vi "Autocycle v0.4.vi"(7 "Message Queue":refnum<queue>, 8 "error in":errorcluster, 10 "All Para":cluster{"Auto Para":T1, "General Para":T2}={"Auto Para"={"Agitator Delays"=[], "TF Delays"=[], "Insertion Delays"=[], "Cutting Delays"=[], "PF Delays"=[], "Measur. Delays"=[], "Reject Delays"=[1000], "BF Delays"=[1000]}, "General Para"={"Max. Cons."=5.0, "Offset 1"=0.0, "Offset 2"=0.0, "Offset 3"=0.0, "Offset 4"=0.0}}) -> (0 "error out":errorcluster)   [LabVIEW 2017]
doc: "v0.3:\n- Added End Cycle & Stop initiated as different stops\n- Make PF & TF not run on the first iteration"
uses:
  support/Message Queue/Message Cluster.ctl
  Controls/Auto Delays.ctl
  support/Controls/General Para.ctl
  Controls/Auto Times.ctl
  Global Variables/RT GV.vi
  Global Variables/FPGA GV.vi
  <vilib>/Utility/error.llb/Error Cluster From Error Code.vi
  <vilib>/rvi/errors/niLvFpgaAdjustHostInterfaceError.vi
  support/Message Queue/Enqueue Message (Single).vi
  <vilib>/rvi/interface/nirviReadWriteControl/nirviReadWriteControl.xnode
  Controls/FPGA Ref.ctl
  NiFpgaLv.dll
  <vilib>/rvi/interface/Simulation/niFpgaSimulationCallBeginRW.vi
  support/Message Queue/Message Queue.lvlib
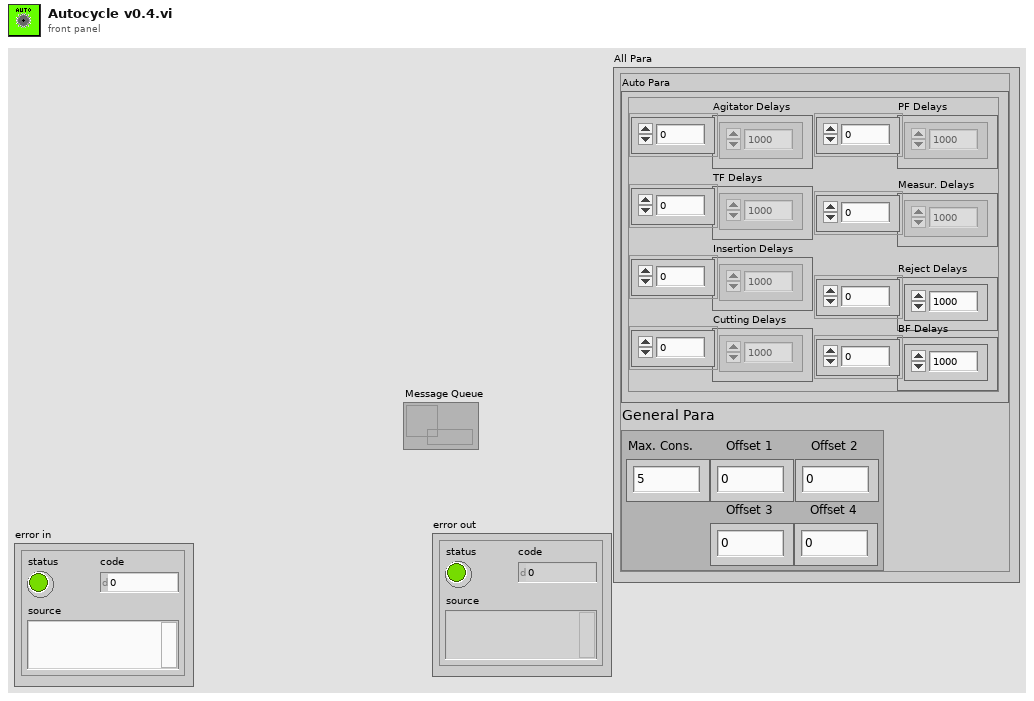
[diagram p1: front panel]
types:
  T1 = typedef "Auto Delays.ctl" = cluster{"Agitator Delays":u32[], "TF Delays":u32[], "Insertion Delays":u32[], "Cutting Delays":u32[], "PF Delays":u32[], "Measur. Delays":dbl[], "Reject Delays":u32[], "BF Delays":u32[]}
  T2 = typedef "General Para.ctl" = cluster{"Max. Cons.":dbl, "Offset 1":dbl, "Offset 2":dbl, "Offset 3":dbl, "Offset 4":dbl}
  T3 = cluster{"Tube Present":bool[], "Output Count":u32}
  T4 = typedef "FPGA Ref.ctl" = refnum<k20>
  T5 = cluster{"TL_Red":bool, "TL_Orange":bool, "TL_Green":bool, "TL_Buzzer":bool, "SOL_Index_Rotary_CW":bool, "SOL_Index_CNVR_Rotary_CCW":bool, "SOL_Index_CNVR_Stopper_Rear":bool, "SOL_Index_CNVR_Output _Separator _Rear":bool, "Bowl Feeder_ ON1":bool, "Pump_CNVR_Motor _ON":bool, "SOL_PC_Gating_CYL_Rear":bool, "SOL_Tube_Feed_Agitatator":bool, "SOL_Tube_Feed_Gating_CYL":bool, "SOL_Insertion _CYL":bool, "SOL_Insertion_Clamp_CYL":bool, "SOL_Cutting_CYL":bool, "SOL_Cutting_Clamp_CYL":bool, "SOL_Insertion_Air_Nozzle":bool, "SOL_Measurement_CYL":bool, "DO1.19":bool, "SOL_Rejection CYL_1":bool, "SOL_Rejection CYL_2":bool, "SOL_Rejection CYL_3":bool, "SOL_Rejection CYL_4":bool, "Bowl Feeder_ON2":bool, "SOL_BF_BlowerON":bool, "SOL_BF1_Track1":bool, "SOL_BF1_Track2":bool, "SOL_BF2_Track1":bool, "SOL_BF2_Track2":bool, "DO1.30":bool, "DO1.31":bool}
  T6 = typedef "Auto Times.ctl" = cluster{"Index Time":u32, "TF Time":u32, "Insertion Time":u32, "Cutting Time":u32, "PF Time":u32, "Meas. Time":u32, "Reject Time":u32}
  T7 = cluster{"Reject 1":bool, "Reject 2":bool, "Reject 3":bool, "Reject 4":bool}
  T8 = cluster{"Tube Present":bool[], "Parts Count":u32}
  T9 = cluster{"seconds since 1Jan1904":timestamp, "Auto Times":T6, "Tube Present":bool[], "Reject Pallets":cluster{"Reject 1":bool, "Reject 2":bool, "Reject 3":bool, "Reject 4":bool}, "Measurements":cluster{"1":dbl, "2":dbl, "3":dbl, "4":dbl}}
  T10 = typedef "Auto Stats.ctl" = cluster{"Time-Stamp":timestamp, "Auto Times":T6, "Measurements":cluster{"1":dbl, "2":dbl, "3":dbl, "4":dbl}, "Outputs":cluster{"Good Parts":u32, "Reject Parts":u32}, "Cycle Time":dbl, "Remarks":string}
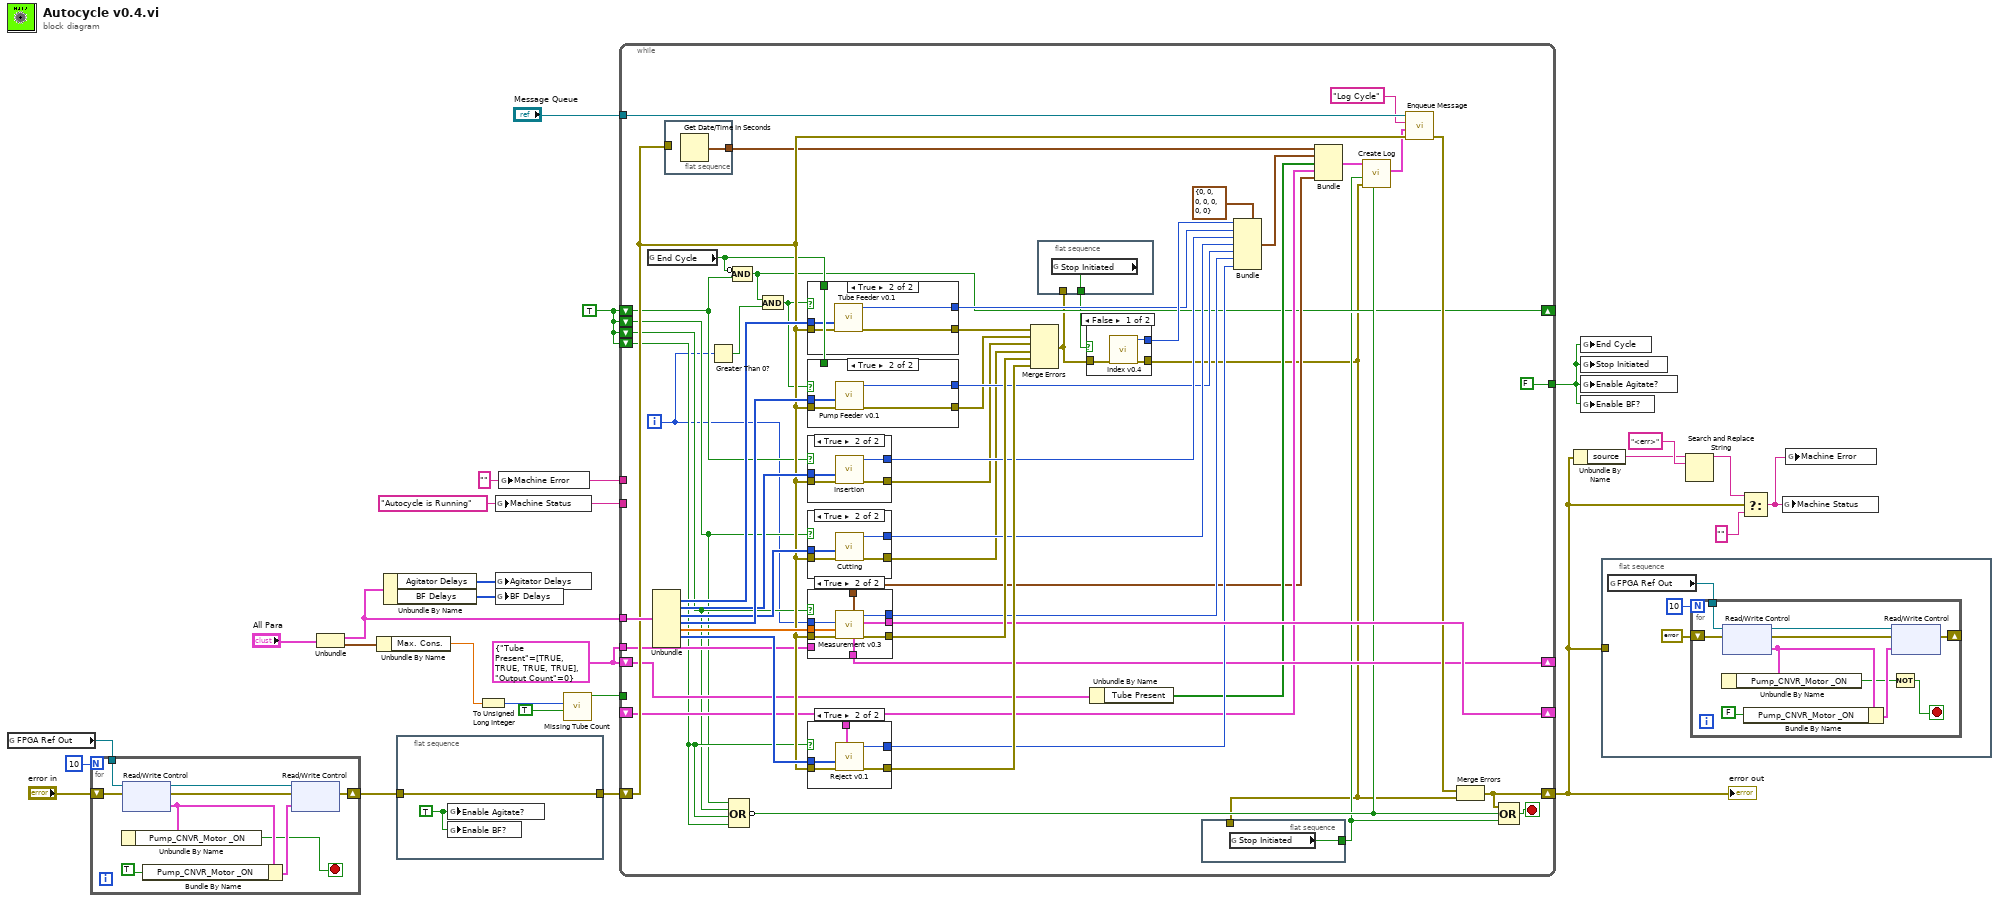
[diagram p0: block diagram]
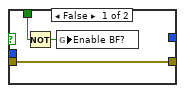
[diagram p3: hidden frame]
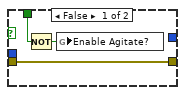
[diagram p6: hidden frame]
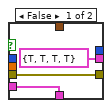
[diagram p8: hidden frame]
diagram:
  w13 = T3 {"Tube Present"=[TRUE, TRUE, TRUE, TRUE], "Output Count"=0} ("Part Count")
  w14 = "" ("Machine Error")
  w21 = "Autocycle is Running" ("Machine Status")
  w7 = TRUE
  n1 = global read "FPGA GV.vi" "FPGA Ref Out"() -> (w24:T4)
  n2 = for {
    N: 10 -> [_]
    tunnel: w24 -> [w35]
    shift-right: [w29] -> w10
    shift-left: "error in" -> [w30]
    stop <- w27 stop-if-true
    n3 = xnode "Read/Write Control"("FPGA VI Reference In"=w35, "error in"=w30) -> ("FPGA VI Reference Out"=w31:T4, "error out"=w32:errorcluster, "DO 1"=w28:T5)
    n4 = Unbundle By Name(w28) -> ("Pump_CNVR_Motor _ON"=w27:bool)
    n5 = Bundle By Name(cluster=w28, "Pump_CNVR_Motor _ON"=TRUE) -> (w34:T5)
    n6 = xnode "Read/Write Control"("FPGA VI Reference In"=w31, "error in"=w32, "DO 1"=w34) -> ("error out"=w29:errorcluster)  [unwired: 1 out]
  }
  n7 = Unbundle("All Para") -> ("Auto Para"=w4:T1, "General Para"=w3:T2)
  n8 = Unbundle By Name(w3) -> ("Max. Cons."=w2:dbl)
  n9 = Unbundle By Name(w4) -> ("Agitator Delays"=w26:u32[], "BF Delays"=w25:u32[])
  n10 = flat-sequence {
    tunnel: [w37] -> w9
    tunnel: w10 -> [w37]
    frame #0 {
      w36 = TRUE ("Enable Agitate?")
      n11 = global write "RT GV.vi" "Enable Agitate?"(w36) -> ()
      n12 = global write "RT GV.vi" "Enable BF?"(w36) -> ()
    }
  }
  n13 = To Unsigned Long Integer(number=w2) -> (unsigned 32bit integer=w1:u32)
  n14 = global write "RT GV.vi" "Machine Status"(w21) -> ()
  n15 = global write "RT GV.vi" "Agitator Delays"(w26) -> ()
  n16 = global write "RT GV.vi" "BF Delays"(w25) -> ()
  n17 = global write "RT GV.vi" "Machine Error"(w14) -> ()
  n18 = call "Missing Tube Count.vi"("ResetMT?"=TRUE, "Max Successive"=w1) -> ("Boolean"=w11:bool)  [unwired: 9 in]
  n19 = while {
    tunnel: w4 -> [w86]
    shift-right: [w63] -> w19
    shift-left: w9 -> [w64]
    shift-right: [w80] -> _
    shift-left: _ -> [w54]
    shift-right: [w45] -> _
    shift-left: w7 -> [w46]
    shift-left: w7 -> [w47]
    shift-left: w7 -> [w48]
    shift-left: w7 -> [w49]
    tunnel: "Message Queue" -> [w70]
    tunnel: [FALSE] -> w6
    tunnel: w21 -> [_]
    tunnel: w14 -> [_]
    shift-right: [w57] -> _
    shift-left: w13 -> [w56]
    tunnel: w13 -> [w58]
    tunnel: w11 -> [_]
    i -> [w41]
    stop <- w79 stop-if-true
    n20 = global read "RT GV.vi" "End Cycle"() -> (w50:bool)
    n21 = Unbundle(w86) -> ("TF Delays"=w89:u32[], "Insertion Delays"=w88:u32[], "Cutting Delays"=w87:u32[], "PF Delays"=w90:u32[], "Measur. Delays"=w84:dbl[], "Reject Delays"=w82:u32[])  [unwired: 2 out]
    n22 = flat-sequence {
      tunnel: w64 -> [_]
      tunnel: [w97] -> w60
      frame #0 {
        n23 = Get Date/Time In Seconds() -> (seconds since 1Jan1904=w97:timestamp)
      }
    }
    n24 = Greater Than 0?(x=w41) -> (x > 0?=w43:bool)
    n25 = Compound Arithmetic op=OR(w47, w48, w49, w49) -> (invert w52:bool)
    n26 = Compound Arithmetic op=AND(invert w50, w46) -> (w45:bool)
    n27 = Compound Arithmetic op=AND(w45, w43) -> (w44:bool)
    n28 = case shown="True" w44 {
      tunnel: w64 -> [w117 w121]
      tunnel: [w117 w120] -> w85
      tunnel: w89 -> [_ w119]
      tunnel: [_ w118] -> w77
      tunnel: w50 -> [w116 _]
      frame False {
        n29 = Not(x=w116) -> (.not. x?=w115:bool)
        n30 = global write "RT GV.vi" "Enable Agitate?"(w115) -> ()
      }
      frame True {
        n31 = call "Tube Feeder v0.1.vi"("error in (no error)"=w121, "TF Para"=w119) -> ("error out"=w120:errorcluster, "TF Time"=w118:u32)  [unwired: 8 in]
      }
    }
    n32 = case shown="True" w44 {
      tunnel: w64 -> [w100 w104]
      tunnel: [w100 w103] -> w66
      tunnel: w90 -> [_ w102]
      tunnel: [_ w101] -> w74
      tunnel: w50 -> [w99 _]
      frame False {
        n33 = Not(x=w99) -> (.not. x?=w98:bool)
        n34 = global write "RT GV.vi" "Enable BF?"(w98) -> ()
      }
      frame True {
        n35 = call "Pump Feeder v0.1.vi"("error in (no error)"=w104, "TF Delays"=w102) -> ("error out"=w103:errorcluster, "PF Time"=w101:u32)  [unwired: 8 in]
      }
    }
    n36 = case shown="True" w46 {
      tunnel: w64 -> [w110 w114]
      tunnel: [w110 w113] -> w67
      tunnel: w88 -> [_ w112]
      tunnel: [_ w111] -> w76
      frame False {
      }
      frame True {
        n37 = call "Insertion.vi"("error in (no error)"=w114, "Insertion Delays"=w112) -> ("error out"=w113:errorcluster, "Insertion Time"=w111:u32)  [unwired: 7 in, 1 out]
      }
    }
    n38 = case shown="True" w47 {
      tunnel: w64 -> [w105 w109]
      tunnel: [w105 w108] -> w68
      tunnel: w87 -> [_ w107]
      tunnel: [_ w106] -> w75
      frame False {
      }
      frame True {
        n39 = call "Cutting.vi"("error in (no error)"=w109, "Cutting Delays"=w107) -> ("error out"=w108:errorcluster, "Cutting Time"=w106:u32)  [unwired: 8 in]
      }
    }
    n40 = case shown="True" w48 {
      tunnel: w64 -> [w130 w138]
      tunnel: [w130 w137] -> w83
      tunnel: w84 -> [_ w136]
      tunnel: [_ w135] -> w73
      tunnel: [_ w134] -> w53
      tunnel: [T7 {"Reject 1"=TRUE, "Reject 2"=TRUE, "Reject 3"=TRUE, "Reject 4"=TRUE} ("Reject Pallets") w133] -> w80
      tunnel: [w128 w132] -> w57
      tunnel: w58 -> [w128 _]
      tunnel: w41 -> [_ w131]
      frame False {
      }
      frame True {
        n41 = call "Measurement v0.3.vi"("error in (no error)"=w138, "TF Delays"=w136, "Loop Count"=w131) -> ("error out"=w137:errorcluster, "Reject Pallets"=w133:T7, "PF Time"=w135:u32, "Part Count"=w132:T8, "Measurements"=w134:cluster{"1":dbl, "2":dbl, "3":dbl, "4":dbl})  [unwired: 4 in]
      }
    }
    n42 = case shown="True" w49 {
      tunnel: w64 -> [w122 w127]
      tunnel: [w122 w126] -> w81
      tunnel: w82 -> [_ w125]
      tunnel: [_ w124] -> w72
      tunnel: w54 -> [_ w123]
      frame False {
      }
      frame True {
        n43 = call "Reject v0.1.vi"("Reject Pallets"=w123, "error in (no error)"=w127, "TF Delays"=w125) -> ("error out"=w126:errorcluster, "PF Time"=w124:u32)  [unwired: 7 in]
      }
    }
    n44 = Merge Errors(w85, w66, w67, w68, w83, w81) -> (w38:errorcluster)
    n45 = flat-sequence {
      tunnel: [w91] -> w39
      tunnel: w38 -> [_]
      frame #0 {
        n46 = global read "RT GV.vi" "Stop Initiated"() -> (w91:bool)
      }
    }
    n47 = case shown="False" w39 {
      tunnel: [w94 _] -> w78
      tunnel: w38 -> [w93 w95]
      tunnel: [w92 w95] -> w40
      frame False {
        n48 = call "Index v0.4.vi"("error in (no error)"=w93) -> ("error out"=w92:errorcluster, "Index Time"=w94:u32)  [unwired: 7 in, 2 out]
      }
      frame True {
      }
    }
    n49 = Unbundle By Name(w56) -> ("Tube Present"=w55:bool[])
    n50 = flat-sequence {
      tunnel: [w96] -> w42
      tunnel: w40 -> [_]
      frame #0 {
        n51 = global read "RT GV.vi" "Stop Initiated"() -> (w96:bool)
      }
    }
    n52 = Bundle(cluster=T6 {"Index Time"=0, "TF Time"=0, "Insertion Time"=0, "Cutting Time"=0, "PF Time"=0, "Meas. Time"=0, "Reject Time"=0} ("Auto Times"), "Index Time"=w78, "TF Time"=w77, "Insertion Time"=w76, "Cutting Time"=w75, "PF Time"=w74, "Meas. Time"=w73, "Reject Time"=w72) -> (w59:T6)
    n53 = Bundle("seconds since 1Jan1904"=w60, "Auto Times"=w59, "Tube Present"=w55, "Reject Pallets"=w54, "Measurements"=w53) -> (w51:T9)  [unwired: 1 in]
    n54 = call "Create Log.vi"("End Cycle?"=w52, "Error in"=w40, "Stop Initiated?"=w42, "Log Input Data"=w51) -> ("Auto Stats"=w61:T10)  [unwired: 7 in]
    n55 = call-poly "Enqueue Message.vi"("error in (no error)"=w64, "Message Data"=w61, "Message"="Log Cycle", "Message Queue"=w70) -> ("error out"=w62:errorcluster)  [unwired: 6 in, 1 out]
    n56 = Merge Errors(w62, w40) -> (w63:errorcluster)
    n57 = Compound Arithmetic op=OR(w63, w52, w42) -> (w79:bool)
  }
  "error out" <- w19
  n58 = Unbundle By Name(w19) -> ("source"=w17:string)
  n59 = global write "RT GV.vi" "End Cycle"(w6) -> ()
  n60 = global write "RT GV.vi" "Stop Initiated"(w6) -> ()
  n61 = global write "RT GV.vi" "Enable Agitate?"(w6) -> ()
  n62 = global write "RT GV.vi" "Enable BF?"(w6) -> ()
  n63 = flat-sequence {
    tunnel: w19 -> [_]
    frame #0 {
      n64 = global read "FPGA GV.vi" "FPGA Ref Out"() -> (w140:T4)
      n65 = for {
        N: 10 -> [_]
        tunnel: w140 -> [w151]
        shift-right: [w145] -> _
        shift-left: errorcluster {"status"=FALSE, "code"=0, "source"=""} ("error out") -> [w146]
        stop <- w142 stop-if-true
        n66 = xnode "Read/Write Control"("FPGA VI Reference In"=w151, "error in"=w146) -> ("FPGA VI Reference Out"=w147:T4, "error out"=w148:errorcluster, "DO 1"=w144:T5)
        n67 = Unbundle By Name(w144) -> ("Pump_CNVR_Motor _ON"=w143:bool)
        n68 = Bundle By Name(cluster=w144, "Pump_CNVR_Motor _ON"=FALSE) -> (w150:T5)
        n69 = Not(x=w143) -> (.not. x?=w142:bool)
        n70 = xnode "Read/Write Control"("FPGA VI Reference In"=w147, "error in"=w148, "DO 1"=w150) -> ("error out"=w145:errorcluster)  [unwired: 1 out]
      }
    }
  }
  n71 = Search and Replace String(input string=w17, search string="<err>") -> (result string=w16:string)  [unwired: 6 in, 3 out]
  n72 = Select(t=w16, s=w19, f="" ("Machine Status")) -> (s? t:f=w15:string)
  n73 = global write "RT GV.vi" "Machine Status"(w15) -> ()
  n74 = global write "RT GV.vi" "Machine Error"(w15) -> ()
